vi "open_spectrometer-v2.vi"(8 "error in":errorcluster, 11 "VISA Refnum in":refnum<visa-resource-name>) -> (0 "error out":errorcluster, 3 "VISA Refnum out":refnum<visa-resource-name>)   [LabVIEW 2021]
doc: "André Romero - 2024\nandretec@ifsc.usp.br"
uses:
  Global_v20.vi
  <instrlib>/Ocean Optics 2000 4000/Ocean Optics 2000 4000.lvlib
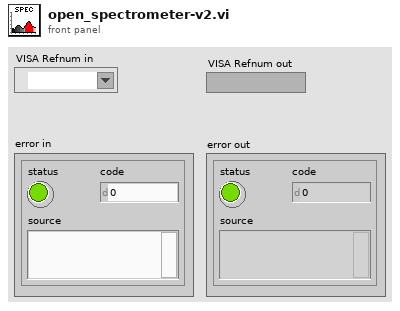
[diagram p1: front panel]
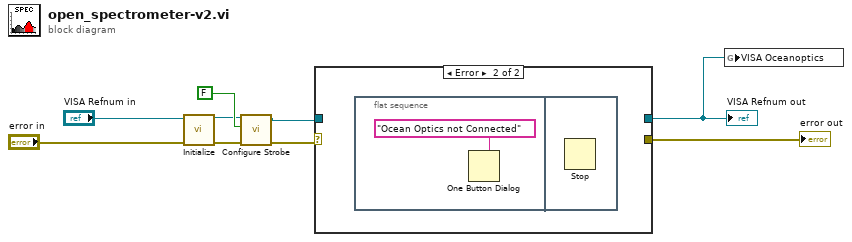
[diagram p0: block diagram]
diagram:
  n1 = call <instrlib>:"Initialize.vi"("error in (no error)"="error in", "VISA resource name"="VISA Refnum in") -> ("error out"=w3:errorcluster, "VISA resource name out"=w2:refnum<visa-resource-name>)  [unwired: 1 in, 7 out]
  n2 = call <instrlib>:"Configure Strobe.vi"("error in (no error)"=w3, "Enable Strobe (Disabled)"=FALSE, "VISA resource name"=w2) -> ("error out"=w7:errorcluster, "VISA resource name out"=w6:refnum<visa-resource-name>)  [unwired: 7 out]
  n3 = case shown="Error" w7 {
    selector: w7 -> [w10 _]
    tunnel: w6 -> [w11 _]
    tunnel: [w11 _] -> w9
    tunnel: [w10 _] -> w8
    frame No Error {
    }
    frame Error {
      n4 = flat-sequence {
        frame #0 {
          n5 = One Button Dialog(message="Ocean Optics not Connected") -> ()  [unwired: 1 in, 1 out]
        }
        frame #1 {
          n6 = Stop() -> ()  [unwired: 1 in]
        }
      }
    }
  }
  "VISA Refnum out" <- w9
  "error out" <- w8
  n7 = global write "Global_v20.vi" "VISA Oceanoptics"(w9) -> ()
